vi "overlayGUI.vi"() -> ()   [LabVIEW 2010]
uses:
  common/enumerations/pixel_lookup_mode_enum.ctl
  common/classes/ImageCollection/ImageCollection/ImageCollection.lvclass
  common/classes/ImageCollection/ImageCollection/position_channels_cluster.ctl
  common/classes/ImageCollection/ImageCollection/pixel_position_cluster.ctl
  common/classes/Image/Image/Image.lvclass
  common/classes/Image/Image/position_channels_cluster.ctl
  RoiGeneric/RoiGeneric.lvclass
  <vilib>/vision/Image Controls.llb/IMAQ Image.ctl
panel:
  in  "Draw ROI":bool
  in  "width":i32(slide)=4 scale=0.0..10.0
  in  "length":i32(slide)=4 scale=0.0..10.0
  in  "ROI":i32
  in  "depth":dbl(slide)=10.0 scale=0.0..10.0
  out "roi":i32[][](array[numeric])
  in  "pixel look-up mode":T1
  out "progress":u8(slide) scale=0.0..100.0
  in  "loadLineDataButton":bool
  in  "loadReferenceStackButton":bool
  in  "ref stack frame":i32(slide) caption="frame" scale=0.0..9.0
  in  "line":i32(slide) scale=0.0..2559.0
  in  "quit":bool
  in  "save":bool
  in  "clear ROIs":bool
  out "line scan image data":T2(plugin-control)
  out "reference stack":T2(plugin-control)
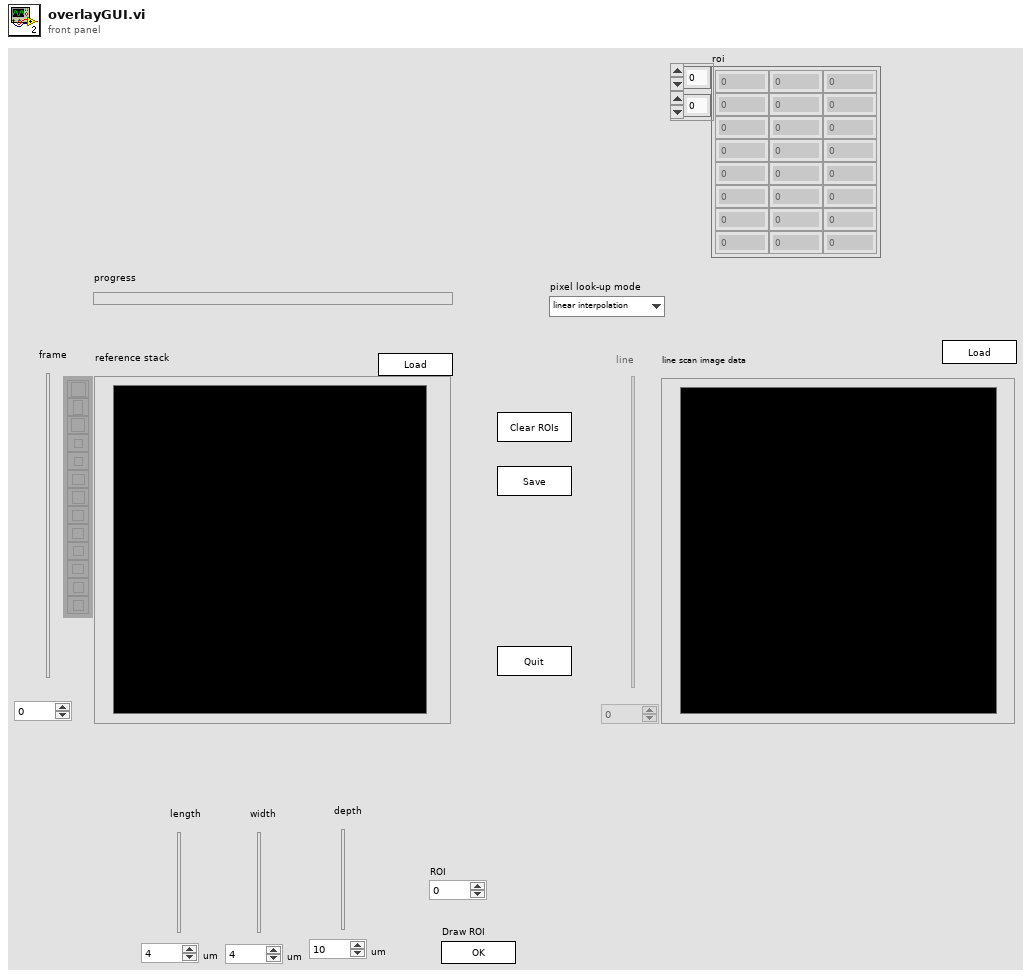
[diagram p1: front panel]
types:
  T1 = typedef "pixel_lookup_mode_enum.ctl" = enum16{"linear interpolation", "binary search"}
  T2 = typedef "IMAQ Image.ctl" = refnum<image>
  T3 = typedef "Image.lvclass/position_channels_cluster.ctl" = cluster{"x":refnum<class "Image.lvclass">, "y":refnum<class "Image.lvclass">, "z":refnum<class "Image.lvclass">}
  T4 = typedef "ImageCollection.lvclass/pixel_position_cluster.ctl" = cluster{"x":dbl, "y":dbl, "z ":dbl}
  T5 = typedef "ImageCollection.lvclass/position_channels_cluster.ctl" = cluster{"x":refnum<class "ImageCollection.lvclass">, "y":refnum<class "ImageCollection.lvclass">, "z":refnum<class "ImageCollection.lvclass">}
  T6 = enum8{"Enabled", "Disabled", "Disabled and Grayed Out"}
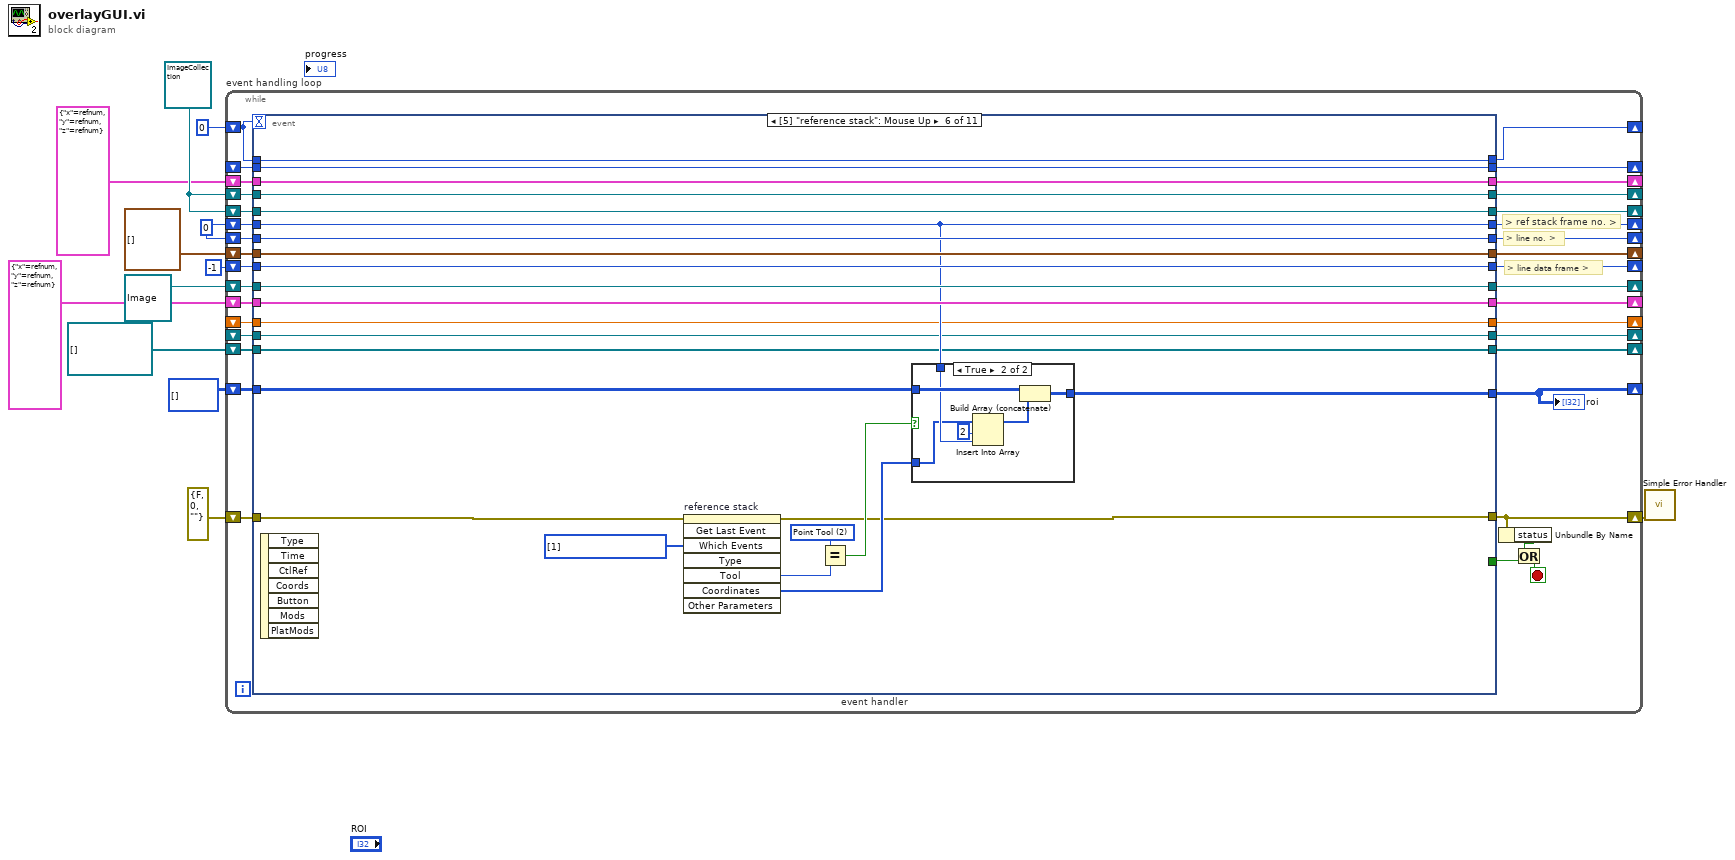
[diagram p0: block diagram]
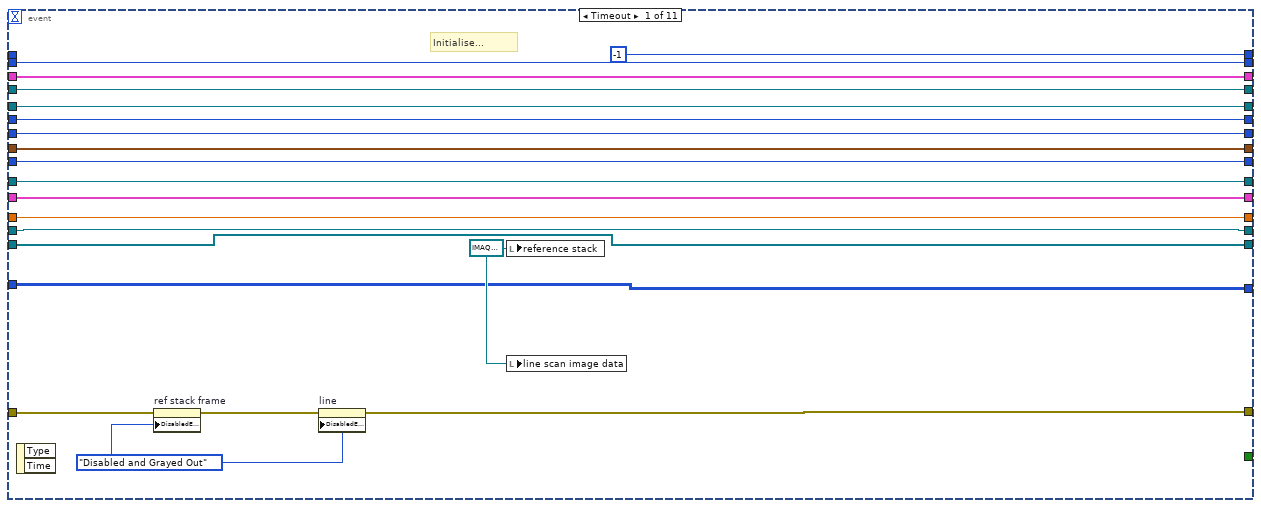
[diagram p2: hidden frame]
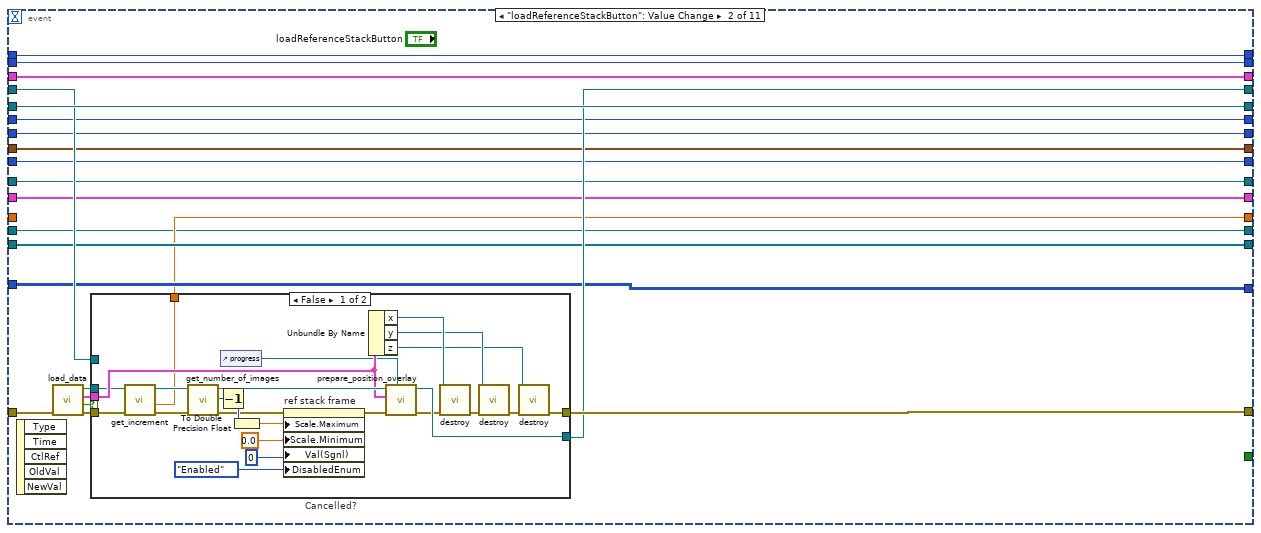
[diagram p3: hidden frame]
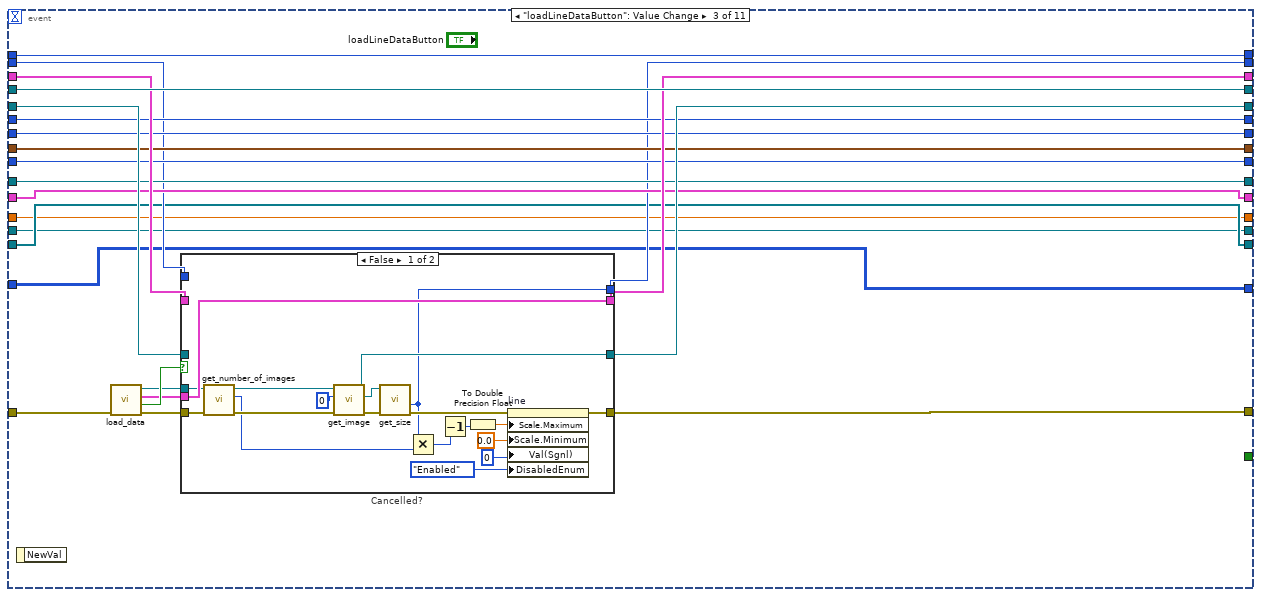
[diagram p5: hidden frame]
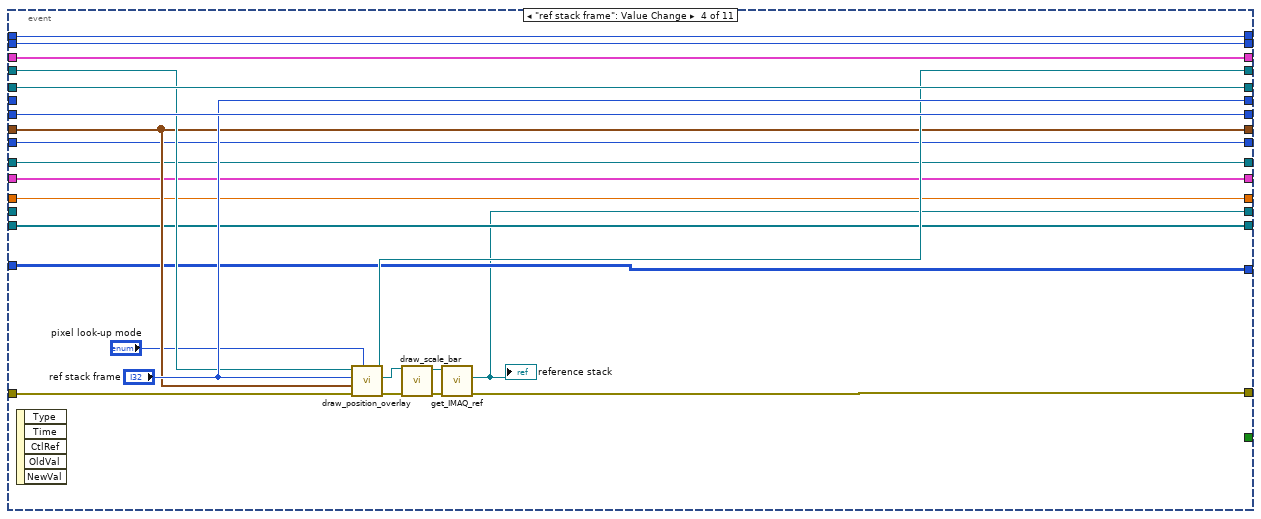
[diagram p7: hidden frame]
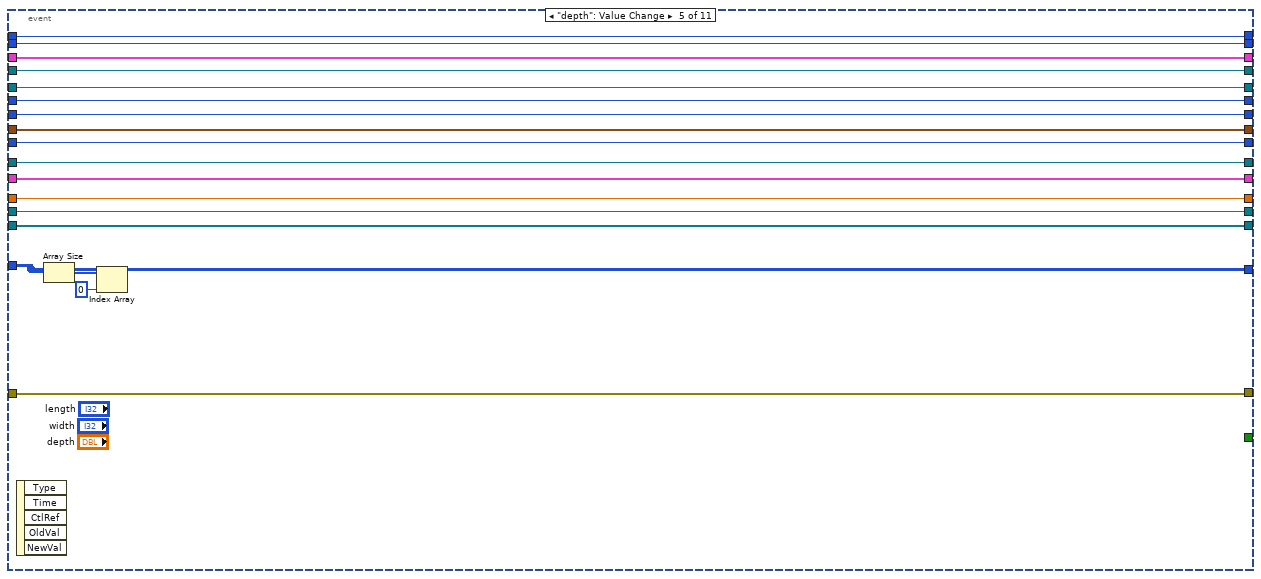
[diagram p8: hidden frame]
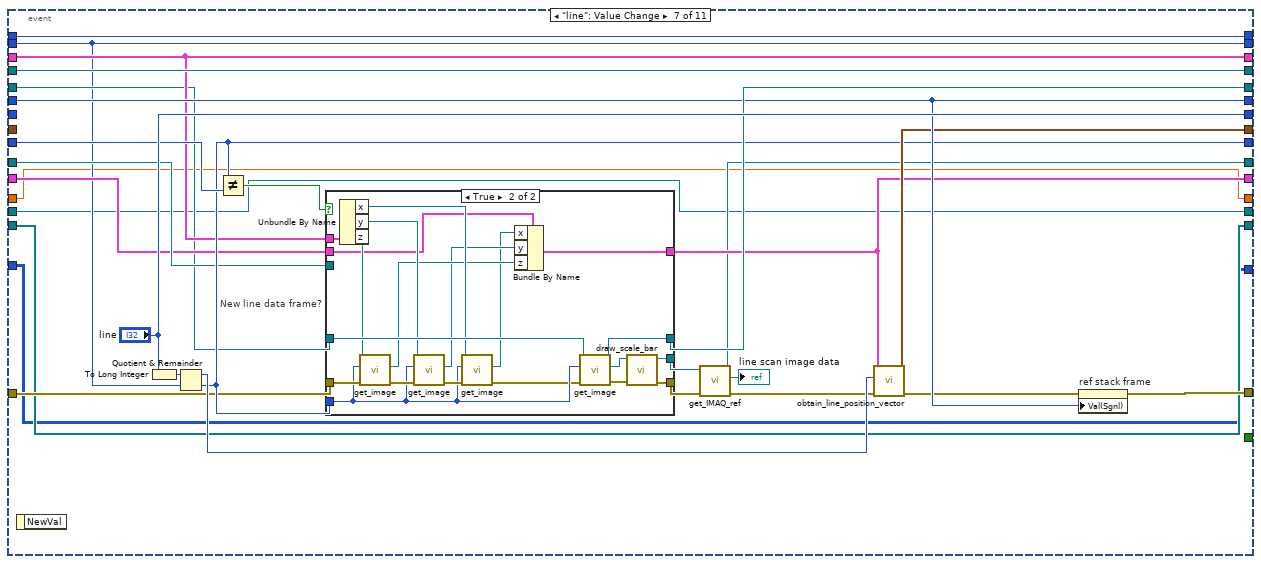
[diagram p10: hidden frame]
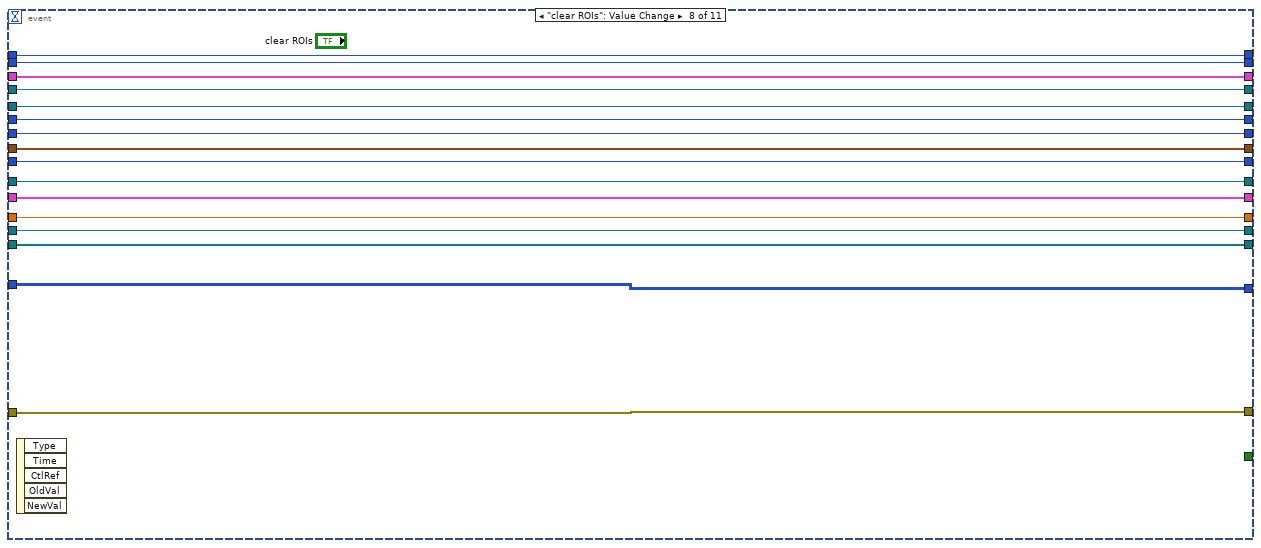
[diagram p12: hidden frame]
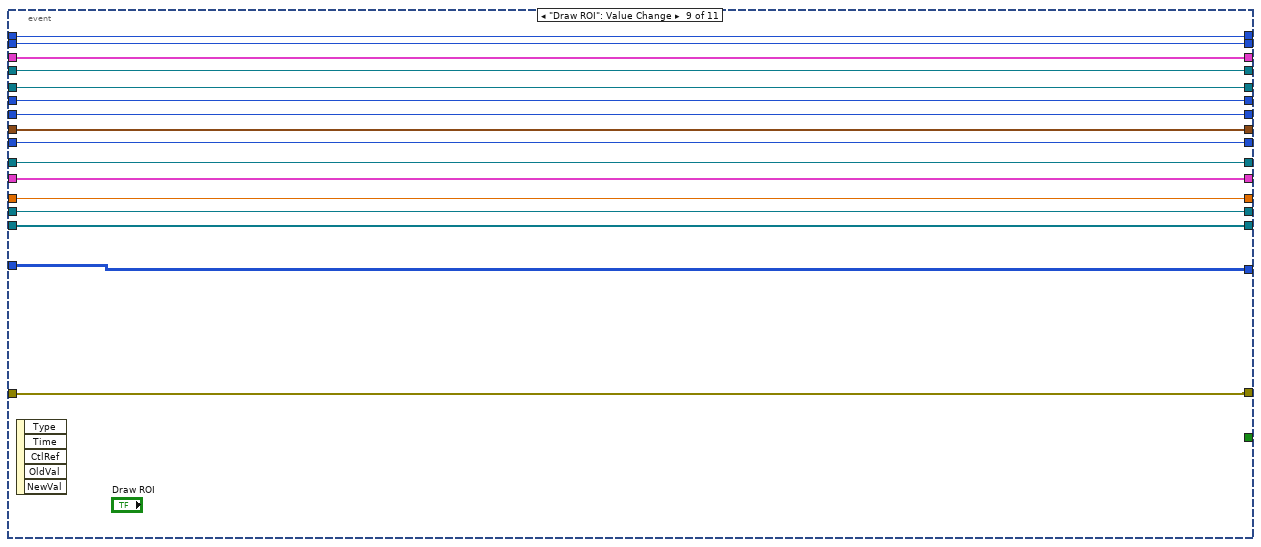
[diagram p13: hidden frame]
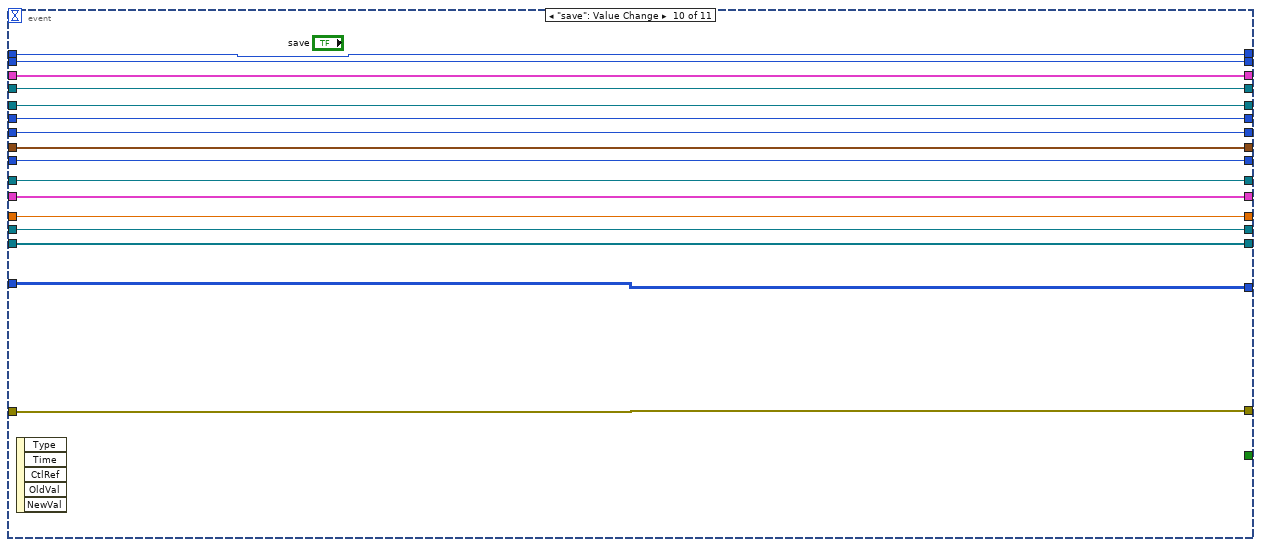
[diagram p14: hidden frame]
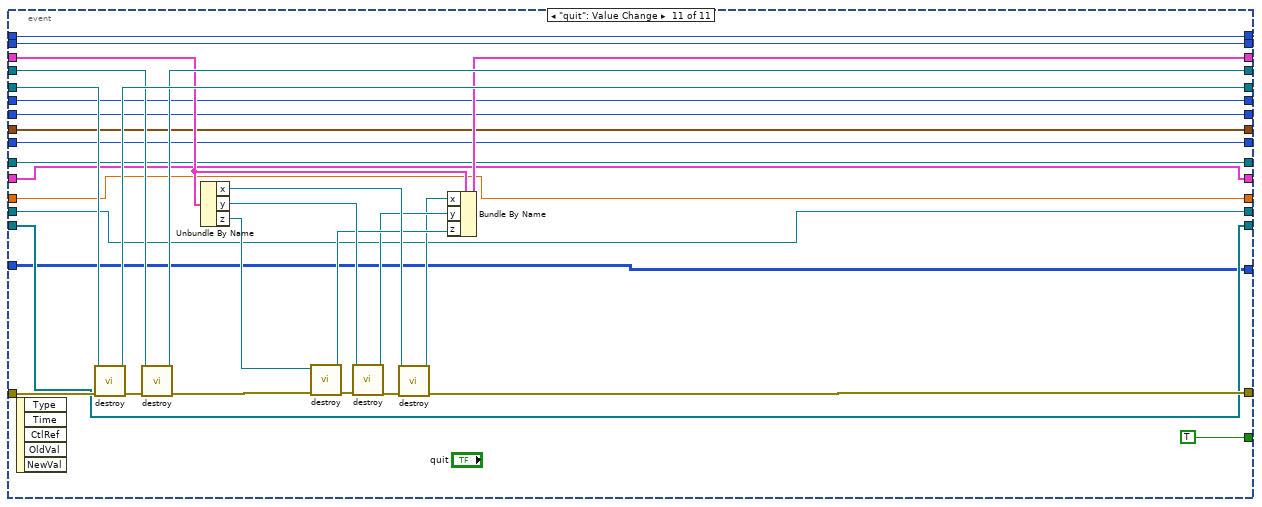
[diagram p15: hidden frame]
diagram:
  w7 = 0
  w11 = refnum<class "ImageCollection.lvclass"> refnum ("ImageCollection.lvclass")
  n1 = while "event handling loop" {
    shift-right: [w46] -> _
    shift-left: w11 -> [w47]
    shift-right: [w44] -> _
    shift-left: w11 -> [w45]
    shift-right: [w40] -> _
    shift-left: 0 -> [w39]
    shift-right: [w38] -> w9
    shift-left: errorcluster {"status"=FALSE, "code"=0, "source"=""} ("error in") -> [w31]
    shift-right: [w36] -> _
    shift-left: T5 {"x"=refnum, "y"=refnum, "z"=refnum} ("Cluster") -> [w37]
    shift-right: [w33] -> _
    shift-left: w7 -> [w35]
    shift-right: [w32] -> _
    shift-left: w7 -> [w34]
    shift-right: [w30] -> _
    shift-left: T4[] [] ("pixel positions") -> [w29]
    shift-right: [w28] -> _
    shift-left: -1 -> [w27]
    shift-right: [w23] -> _
    shift-left: refnum<class "Image.lvclass"> refnum ("Image.lvclass") -> [w26]
    shift-right: [w24] -> _
    shift-left: T3 {"x"=refnum, "y"=refnum, "z"=refnum} ("position channels") -> [w25]
    shift-right: [w22] -> _
    shift-left: _ -> [w21]
    shift-right: [w19] -> _
    shift-left: refnum<class "RoiGeneric.lvclass">[] [] -> [w20]
    shift-right: [w17] -> _
    shift-left: i32[][] [] -> [w18]
    shift-right: [w16] -> _
    shift-left: _ -> [w15]
    shift-right: [w14] -> _
    shift-left: _ -> [w13]
    stop <- w41 stop-if-true
    # "> ref stack frame no. >"
    # "> line no. >"
    # "> line data frame >"
    n2 = event "event handler" shown="[5] \"reference stack\": Mouse Up" {
      selector: _ -> [_ _ _ _ _ _ _ _ _ _ _]
      dyn-events: _ -> [_ _ _ _ _ _ _ _ _ _ _]
      timeout: w39 -> [_ _ _ _ _ _ _ _ _ _ _]
      tunnel: w47 -> [w66 w82 w138 w179 w203 w226 w258 w302 w318 w334 w363]
      tunnel: [w66 w80 w138 w178 w203 w226 w258 w302 w318 w334 w362] -> w46
      tunnel: w45 -> [w65 w88 w135 w184 w202 w225 w239 w301 w317 w333 w365]
      tunnel: [w65 w88 w132 w184 w202 w225 w259 w301 w317 w333 w364] -> w44
      tunnel: [_ _ _ _ _ _ _ _ _ _ TRUE] -> w42
      tunnel: [-1 w89 w139 w185 w201 w224 w262 w298 w316 w330 w359] -> w40
      tunnel: w39 -> [_ w89 w139 w185 w201 w224 w262 w298 w316 w330 w359]
      tunnel: [w58 w85 w128 w170 w186 w207 w257 w300 w303 w332 w356] -> w38
      tunnel: w37 -> [w64 w79 w134 w183 w200 w223 w241 w299 w315 w331 w349]
      tunnel: [w64 w79 w133 w183 w200 w223 w241 w299 w315 w331 w348] -> w36
      tunnel: w35 -> [w61 w77 w126 _ w188 w209 w256 w296 w305 w328 w345]
      tunnel: w34 -> [w60 w78 w127 w182 w199 w222 _ w297 w314 w329 w346]
      tunnel: [w61 w77 w126 "ref stack frame" w188 w209 w256 w296 w305 w328 w345] -> w33
      tunnel: [w60 w78 w127 w182 w199 w222 "line" w297 w314 w329 w346] -> w32
      tunnel: w31 -> [w63 w87 w137 w181 w186 w208 w240 w300 w303 w332 w361]
      tunnel: [w57 w76 w125 w177 w198 w221 w254 w295 w313 w327 w343] -> w30
      tunnel: w29 -> [w57 w76 w125 w177 w198 w221 _ w295 w313 w327 w343]
      tunnel: [w56 w75 w124 w176 w197 w220 w251 w294 w312 w326 w342] -> w28
      tunnel: w27 -> [w56 w75 w124 w176 w197 w220 w252 w294 w312 w326 w342]
      tunnel: w26 -> [w55 w74 w123 w175 w195 w218 w249 w293 w310 w325 w341]
      tunnel: w25 -> [w54 w73 w122 w174 w196 w219 w244 w292 w311 w324 w340]
      tunnel: [w54 w73 w122 w174 w196 w219 w243 w292 w311 w324 w340] -> w24
      tunnel: [w55 w74 w123 w175 w195 w218 w242 w293 w310 w325 w341] -> w23
      tunnel: [w52 w72 w121 w173 w194 w217 w238 w291 w309 w323 w339] -> w22
      tunnel: w21 -> [w52 w72 w120 w173 w194 w217 w238 w291 w309 w323 w339]
      tunnel: [w51 w71 w119 w171 w193 w206 w237 w290 w308 w322 w338] -> w19
      tunnel: w20 -> [w51 w71 w119 w171 w193 w206 w237 w290 w308 w322 w338]
      tunnel: w18 -> [w50 w70 w118 w165 w190 w211 w236 w289 w304 w321 w337]
      tunnel: [w50 w70 w118 w165 w190 w210 w236 w289 w304 w321 w337] -> w17
      tunnel: [w49 w69 w117 w164 w189 w205 w235 w288 w307 w320 w336] -> w16
      tunnel: w15 -> [w49 _ w117 w164 w189 w205 w235 w288 w307 w320 w336]
      tunnel: [w48 w68 w116 w163 w187 w204 w234 w287 w306 w319 w335] -> w14
      tunnel: w13 -> [w48 w68 w116 _ w187 w204 w234 w287 w306 w319 w335]
      event Timeout {
        w53 = T2 refnum ("reference stack")
        w59 = T6."Disabled and Grayed Out" ("Disabled")
        # "Initialise..."
        n3 = event-data() -> ()  [unwired: 1 in, 2 out]
        n4 = property on="ref stack frame" class="Slide (strict)"(error in=w63, "DisabledEnum"=w59) -> (error out=w62:errorcluster)  [unwired: 1 in, 1 out]
        n5 = property on="line" class="Slide (strict)"(error in=w62, "DisabledEnum"=w59) -> (error out=w58:errorcluster)  [unwired: 1 in, 1 out]
        n6 = local write "reference stack"(w53) -> ()
        n7 = local write "line scan image data"(w53) -> ()
      }
      event "loadReferenceStackButton": Value Change {
        n8 = event-data() -> ()  [unwired: 1 in, 5 out]
        n9 = call "load_data.vi"("error in (no error)"=w87) -> ("error out"=w86:errorcluster, "cancelled?"=w84:bool, "position feedback"=w83:T5, "ImageCollection.lvclass"=w81:refnum<class "ImageCollection.lvclass">)  [unwired: 7 in]
        n10 = case "Cancelled?" shown="False" w84 {
          tunnel: w86 -> [w94 w115]
          tunnel: [w99 w115] -> w85
          tunnel: w83 -> [w103 _]
          tunnel: w82 -> [_ w114]
          tunnel: w81 -> [w93 _]
          tunnel: [w104 w114] -> w80
          tunnel: [w90 _] -> w69
          frame False {
            n11 = call "get_increment.vi"("error in (no error)"=w94, "ImageCollection in"=w93) -> ("error out"=w91:errorcluster, "z increment"=w90:dbl[unit], "ImageCollection out"=w92:refnum<class "ImageCollection.lvclass">)  [unwired: 5 in, 2 out]
            n12 = call-dynamic "get_number_of_images.vi"("error in (no error)"=w91, "ImageCollection in"=w92) -> ("error out"=w107:errorcluster, "size"=w110:i32, "ImageCollection out"=w105:refnum<class "ImageCollection.lvclass">)  [unwired: 7 in]
            n13 = Decrement(x=w110) -> (x-1=w111:i32)
            n14 = control-ref of="progress"() -> (w95:refnum<vi>)
            n15 = To Double Precision Float(number=w111) -> (double precision float=w109:dbl)
            n16 = property on="ref stack frame" class="Slide (strict)"(error in=w107, "Scale.Maximum"=w109, "Scale.Minimum"=0.0 ("Scale.Range:Minimum"), "Val(Sgnl)"=0 ("Value (Signaling)"), "DisabledEnum"=T6."Enabled" ("Disabled")) -> (error out=w106:errorcluster)  [unwired: 1 in, 1 out]
            n17 = Unbundle By Name(w103) -> ("x"=w98:refnum<class "ImageCollection.lvclass">, "y"=w97:refnum<class "ImageCollection.lvclass">, "z"=w96:refnum<class "ImageCollection.lvclass">)
            n18 = call "prepare_position_overlay.vi"("progress bar ref"=w95, "error in (no error)"=w106, "position channels"=w103, "ImageCollection in"=w105) -> ("error out"=w100:errorcluster, "ImageCollection out"=w104:refnum<class "ImageCollection.lvclass">)  [unwired: 5 in, 1 out]
            n19 = call-dynamic "destroy.vi"("error in (no error)"=w100, "ImageCollection in"=w98) -> ("error out"=w102:errorcluster)  [unwired: 8 in, 1 out]
            n20 = call-dynamic "destroy.vi"("error in (no error)"=w102, "ImageCollection in"=w97) -> ("error out"=w101:errorcluster)  [unwired: 8 in, 1 out]
            n21 = call-dynamic "destroy.vi"("error in (no error)"=w101, "ImageCollection in"=w96) -> ("error out"=w99:errorcluster)  [unwired: 8 in, 1 out]
          }
          frame True {
          }
        }
      }
      event "loadLineDataButton": Value Change {
        n22 = event-data() -> ()  [unwired: 1 in, 1 out]
        n23 = call "load_data.vi"("error in (no error)"=w137) -> ("error out"=w129:errorcluster, "cancelled?"=w136:bool, "position feedback"=w130:T5, "ImageCollection.lvclass"=w131:refnum<class "ImageCollection.lvclass">)  [unwired: 7 in]
        n24 = case "Cancelled?" shown="False" w136 {
          tunnel: w135 -> [_ w162]
          tunnel: [w144 w162] -> w132
          tunnel: w134 -> [_ w161]
          tunnel: [w158 w161] -> w133
          tunnel: w131 -> [w151 _]
          tunnel: w130 -> [w158 _]
          tunnel: w129 -> [w152 w160]
          tunnel: [w153 w160] -> w128
          tunnel: [w140 w159] -> w121
          tunnel: w120 -> [_ w159]
          frame False {
            n25 = call-dynamic "get_number_of_images.vi"("error in (no error)"=w152, "ImageCollection in"=w151) -> ("error out"=w149:errorcluster, "size"=w142:i32, "ImageCollection out"=w147:refnum<class "ImageCollection.lvclass">)  [unwired: 7 in]
            n26 = call-dynamic "get_image.vi"("error in (no error)"=w149, "index"=0, "ImageCollection in"=w147) -> ("error out"=w146:errorcluster, "Image.lvclass"=w143:refnum<class "Image.lvclass">, "ImageCollection out"=w144:refnum<class "ImageCollection.lvclass">)  [unwired: 6 in]
            n27 = call-dynamic "get_size.vi"("error in (no error)"=w146, "Image in"=w143) -> ("error out"=w145:errorcluster, "y resolution"=w140:i32)  [unwired: 2 in, 6 out]
            n28 = Multiply(x=w140, y=w142) -> (x*y=w141:i32)
            n29 = Decrement(x=w141) -> (x-1=w150:i32)
            n30 = To Double Precision Float(number=w150) -> (double precision float=w155:dbl)
            n31 = property on="line" class="Slide (strict)"(error in=w145, "Scale.Maximum"=w155, "Scale.Minimum"=0.0 ("Scale.Range:Minimum"), "Val(Sgnl)"=0 ("Value (Signaling)"), "DisabledEnum"=T6."Enabled" ("Disabled")) -> (error out=w153:errorcluster)  [unwired: 1 in, 1 out]
          }
          frame True {
          }
        }
      }
      event "ref stack frame": Value Change {
        n32 = event-data() -> ()  [unwired: 1 in, 5 out]
        n33 = call "draw_position_overlay.vi"("pixel look-up mode"="pixel look-up mode", "error in (no error)"=w181, "pixel positions"=w177, "frame index"="ref stack frame", "ImageCollection in"=w179) -> ("error out"=w167:errorcluster, "Image.lvclass"=w166:refnum<class "Image.lvclass">, "ImageCollection out"=w178:refnum<class "ImageCollection.lvclass">)  [unwired: 4 in]
        n34 = call "draw_scale_bar.vi"("error in (no error)"=w167, "Image in"=w166) -> ("error out"=w168:errorcluster, "Image out"=w169:refnum<class "Image.lvclass">)  [unwired: 8 in]
        n35 = call-dynamic "get_IMAQ_ref.vi"("error in (no error)"=w168, "Image.lvclass in"=w169) -> ("error out"=w170:errorcluster, "Image"=w163:T2)  [unwired: 5 in, 3 out]
        "reference stack" <- w163
      }
      event "depth": Value Change {
        n36 = event-data() -> ()  [unwired: 1 in, 5 out]
        n37 = Array Size(array=w190) -> (size(s)=w192:i32[])
        n38 = Index Array(array=w192, index=0) -> ()  [unwired: 1 out]
      }
      event "reference stack": Mouse Up {
        w214 = 2 items=["None", "Selection Tool", "Point Tool", "Line Tool", "Rectangle Tool", "Oval Tool", "Polygon Tool", "ClosedFreehandTool", "Annulus Tool", "Rotated Rectangle Tool", "Zoom Tool", "Pan Tool", "Polyline Tool", "Freehand Tool"] ("Tool")
        w216 = i32[] [1] items=["No  event", "Click event", "Draw event", "Move event", "Size event", "Scroll event", "Activate event", "Close event", "Double click event"] ("Events list (all)")
        n39 = event-data() -> ()  [unwired: 1 in, 7 out]
        n40 = invoke on="reference stack" class="ImageControl" method="Get Last Event"(error in=w208, "Which Events"=w216) -> (error out=w207:errorcluster, "Tool"=w215:i32, "Coordinates"=w212:i32[])  [unwired: 6 in, 5 out]
        n41 = Equal?(x=w214, y=w215) -> (x = y?=w213:bool)
        n42 = case shown="True" w213 {
          tunnel: w212 -> [_ w228]
          tunnel: w211 -> [w227 w233]
          tunnel: [w227 w232] -> w210
          tunnel: w209 -> [_ w230]
          frame False {
          }
          frame True {
            n43 = Insert Into Array(array=w228, index=2, new element=w230) -> (w229:i32[])
            n44 = Build Array (concatenate)(w233, w229) -> (w232:i32[][])
          }
        }
      }
      event "line": Value Change {
        n45 = event-data() -> ()  [unwired: 1 in, 1 out]
        n46 = To Long Integer(number="line") -> (32bit integer=w261:i32)
        n47 = Quotient & Remainder(x=w261, y=w238) -> (x-y*floor(x/y)=w253:i32, floor(x/y)=w251:i32)
        n48 = Not Equal?(x=w251, y=w252) -> (x != y?=w250:bool)
        n49 = case "New line data frame?" shown="True" w250 {
          tunnel: w240 -> [w266 w278]
          tunnel: w239 -> [w265 w284]
          tunnel: [w265 w283] -> w259
          tunnel: [w266 w282] -> w246
          tunnel: w251 -> [_ w273]
          tunnel: w249 -> [w264 _]
          tunnel: [w264 w281] -> w248
          tunnel: w244 -> [w263 w271]
          tunnel: [w263 w267] -> w243
          tunnel: w241 -> [_ w280]
          frame False {
          }
          frame True {
            n50 = Unbundle By Name(w280) -> ("x"=w274:refnum<class "ImageCollection.lvclass">, "y"=w275:refnum<class "ImageCollection.lvclass">, "z"=w279:refnum<class "ImageCollection.lvclass">)
            n51 = call-dynamic "get_image.vi"("error in (no error)"=w278, "index"=w273, "ImageCollection in"=w279) -> ("error out"=w277:errorcluster, "Image.lvclass"=w270:refnum<class "Image.lvclass">)  [unwired: 6 in, 1 out]
            n52 = call-dynamic "get_image.vi"("error in (no error)"=w277, "index"=w273, "ImageCollection in"=w275) -> ("error out"=w276:errorcluster, "Image.lvclass"=w269:refnum<class "Image.lvclass">)  [unwired: 6 in, 1 out]
            n53 = call-dynamic "get_image.vi"("error in (no error)"=w276, "index"=w273, "ImageCollection in"=w274) -> ("error out"=w272:errorcluster, "Image.lvclass"=w268:refnum<class "Image.lvclass">)  [unwired: 6 in, 1 out]
            n54 = Bundle By Name(cluster=w271, "x"=w268, "y"=w269, "z"=w270) -> (w267:T3)
            n55 = call-dynamic "get_image.vi"("error in (no error)"=w272, "index"=w273, "ImageCollection in"=w284) -> ("error out"=w286:errorcluster, "Image.lvclass"=w285:refnum<class "Image.lvclass">, "ImageCollection out"=w283:refnum<class "ImageCollection.lvclass">)  [unwired: 6 in]
            n56 = call "draw_scale_bar.vi"("error in (no error)"=w286, "Image in"=w285) -> ("error out"=w282:errorcluster, "Image out"=w281:refnum<class "Image.lvclass">)  [unwired: 8 in]
          }
        }
        n57 = call-dynamic "get_IMAQ_ref.vi"("error in (no error)"=w246, "Image.lvclass in"=w248) -> ("error out"=w247:errorcluster, "Image"=→"line scan image data":T2, "Image.lvclass out"=w242:refnum<class "Image.lvclass">)  [unwired: 5 in, 2 out]
        n58 = call "obtain_line_position_vector.vi"("error in (no error)"=w247, "line index (relative to frame)"=w253, "position channels"=w243) -> ("error out"=w255:errorcluster, "pixel positions"=w254:T4[])  [unwired: 7 in]
        n59 = property on="ref stack frame" class="Slide (strict)"(error in=w255, "Val(Sgnl)"=w256) -> (error out=w257:errorcluster)  [unwired: 1 in, 1 out]
      }
      event "clear ROIs": Value Change {
        n60 = event-data() -> ()  [unwired: 1 in, 5 out]
      }
      event "Draw ROI": Value Change {
        n61 = event-data() -> ()  [unwired: 1 in, 5 out]
      }
      event "save": Value Change {
        n62 = event-data() -> ()  [unwired: 1 in, 5 out]
      }
      event "quit": Value Change {
        n63 = event-data() -> ()  [unwired: 1 in, 5 out]
        n64 = call-dynamic "destroy.vi"("error in (no error)"=w361, "ImageCollection in"=w365) -> ("error out"=w360:errorcluster, "ImageCollection out"=w364:refnum<class "ImageCollection.lvclass">)  [unwired: 8 in]
        n65 = call-dynamic "destroy.vi"("error in (no error)"=w360, "ImageCollection in"=w363) -> ("error out"=w344:errorcluster, "ImageCollection out"=w362:refnum<class "ImageCollection.lvclass">)  [unwired: 8 in]
        n66 = Unbundle By Name(w349) -> ("x"=w353:refnum<class "ImageCollection.lvclass">, "y"=w354:refnum<class "ImageCollection.lvclass">, "z"=w355:refnum<class "ImageCollection.lvclass">)
        n67 = call-dynamic "destroy.vi"("error in (no error)"=w344, "ImageCollection in"=w355) -> ("error out"=w358:errorcluster, "ImageCollection out"=w352:refnum<class "ImageCollection.lvclass">)  [unwired: 8 in]
        n68 = call-dynamic "destroy.vi"("error in (no error)"=w358, "ImageCollection in"=w354) -> ("error out"=w357:errorcluster, "ImageCollection out"=w351:refnum<class "ImageCollection.lvclass">)  [unwired: 8 in]
        n69 = call-dynamic "destroy.vi"("error in (no error)"=w357, "ImageCollection in"=w353) -> ("error out"=w356:errorcluster, "ImageCollection out"=w350:refnum<class "ImageCollection.lvclass">)  [unwired: 8 in]
        n70 = Bundle By Name(cluster=w349, "x"=w350, "y"=w351, "z"=w352) -> (w348:T5)
      }
    }
    "roi" <- w17
    n71 = Unbundle By Name(w38) -> ("status"=w43:bool)
    n72 = Or(x=w43, y=w42) -> (x .or. y?=w41:bool)
  }
  n73 = call <vilib>:"Simple Error Handler.vi"("error in (no error)"=w9) -> ()  [unwired: 4 in, 5 out]
